vi "fgv.vi"(11 "Function":enum16{"reset", "increase", "decrease"}(ring)) -> (3 "Total":i32)   [LabVIEW 2020]
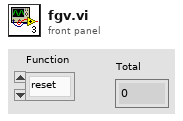
[diagram p1: front panel]
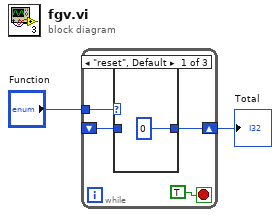
[diagram p0: block diagram]
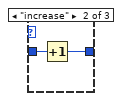
[diagram p2: hidden frame]
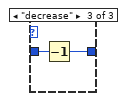
[diagram p3: hidden frame]
diagram:
  n1 = while {
    tunnel: "Function" -> [w6]
    shift-right: [w4] -> w1
    shift-left: _ -> [w5]
    stop <- TRUE stop-if-true
    n2 = case shown="\"reset\", Default" w6 {
      tunnel: [0 w9 w11] -> w4
      tunnel: w5 -> [_ w8 w10]
      frame "reset", Default {
      }
      frame "increase" {
        n3 = Increment(x=w8) -> (x+1=w9:i32)
      }
      frame "decrease" {
        n4 = Decrement(x=w10) -> (x-1=w11:i32)
      }
    }
  }
  "Total" <- w1
